vi "Version_2.0_Single_Column_Code.vi"() -> ()   [LabVIEW 2020] (continued)
                                n6258 = local read "Pause Elution"() -> (w6664:bool)
                                n6259 = case shown="True" w6664 {
                                tunnel: w6663 -> [w6675 _]
                                tunnel: w6671 -> [w6674 w6717]
                                tunnel: w6670 -> [w6673 _]
                                tunnel: w6669 -> [w6672 _]
                                frame False {
                                n6260 = stacked-sequence {
                                tunnel: w6675 -> [_ w6681]
                                tunnel: w6674 -> [_ w6680]
                                tunnel: w6673 -> [_ w6679]
                                tunnel: w6672 -> [_ w6678]
                                frame #0 {
                                n6261 = Wait (ms)(milliseconds to wait=u32 3000) -> ()  [unwired: 1 out]
                                n6262 = local write "Signal"(TRUE ("Signal")) -> ()
                                }
                                frame #1 {
                                n6263 = while {
                                tunnel: w6681 -> [w6693]
                                tunnel: w6680 -> [w6692]
                                tunnel: w6679 -> [w6691]
                                tunnel: w6678 -> [w6690]
                                stop <- w6685 stop-if-true
                                n6264 = stacked-sequence {
                                tunnel: w6693 -> [_ w6700]
                                tunnel: w6692 -> [_ w6699]
                                tunnel: w6691 -> [_ w6698]
                                tunnel: w6690 -> [_ w6697]
                                frame #0 {
                                n6265 = Wait (ms)(milliseconds to wait=u32 500) -> ()  [unwired: 1 out]
                                }
                                frame #1 {
                                n6266 = call "AbsolutePlungerPosition (SubVI).vi"("VISA Refnum in"=w6699) -> ("Plunger Position"=w6696:i32)  [unwired: 10 in]
                                n6267 = case shown="\"High Resolution Pumping\"" w6698 {
                                tunnel: w6700 -> [w6705 w6714]
                                tunnel: w6696 -> [w6706 w6713]
                                tunnel: [w6704 w6711] -> w6695
                                tunnel: w6697 -> [w6703 w6712]
                                frame "Standard Pumping", Default {
                                n6268 = Subtract(x=w6705, y=w6706) -> (x-y=w6702:dbl)
                                n6269 = Absolute Value(x=w6702) -> (abs(x)=w6701:dbl)
                                n6270 = Multiply(x=w6701, y=w6703) -> (x*y=w6708:dbl)
                                n6271 = Divide(x=w6708, y=3000.0) -> (x/y=w6704:dbl)
                                }
                                frame "High Resolution Pumping" {
                                n6272 = Subtract(x=w6714, y=w6713) -> (x-y=w6710:dbl)
                                n6273 = Absolute Value(x=w6710) -> (abs(x)=w6709:dbl)
                                n6274 = Multiply(x=w6709, y=w6712) -> (x*y=w6716:dbl)
                                n6275 = Divide(x=w6716, y=24000.0) -> (x/y=w6711:dbl)
                                }
                                }
                                n6276 = local write "Volume being Injected \nin this process"(w6695) -> ()
                                }
                                }
                                n6277 = local read "Volume being Injected \nin this process"() -> (w6683:dbl)
                                n6278 = local read "Affinity Elution \nGraph Min CutOff"() -> (w6682:dbl)
                                n6279 = local read "Stopper that ends \nthe main loops"() -> (w6688:bool)
                                n6280 = local read "Divert Sample \ninto Column-2"() -> (w6689:bool)
                                n6281 = Greater Or Equal?(x=w6683, y=w6682) -> (x >= y?=w6684:bool)
                                n6282 = Or(x=w6689, y=w6688) -> (x .or. y?=w6686:bool)
                                n6283 = local read "Pause Elution"() -> (w6687:bool)
                                n6284 = local write "Affinity Elution \nis Approaching"(w6684) -> ()
                                n6285 = Or(x=w6687, y=w6686) -> (x .or. y?=w6685:bool)
                                }
                                }
                                }
                                }
                                frame True {
                                n6286 = stacked-sequence {
                                tunnel: w6717 -> [_ w6720 _]
                                frame #0 {
                                n6287 = Wait (ms)(milliseconds to wait=u32 2000) -> ()  [unwired: 1 out]
                                }
                                frame #1 {
                                n6288 = local read "Signal"() -> (w6719:bool)
                                n6289 = case shown="True" w6719 {
                                tunnel: w6720 -> [_ w6726]
                                frame False {
                                }
                                frame True {
                                n6290 = local read "Volume being Injected \nin this process"() -> (w6724:dbl)
                                n6291 = local read "Net Elution \nVolume"() -> (w6723:dbl)
                                n6292 = local write "Signal"(FALSE ("Signal")) -> ()
                                n6293 = Add(x=w6724, y=w6723) -> (x+y=w6722:dbl)
                                n6294 = call "AbsolutePlungerPosition (SubVI).vi"("VISA Refnum in"=w6726) -> ("Plunger Position"=w6725:i32)  [unwired: 10 in]
                                n6295 = local write "Net Elution \nVolume"(w6722) -> ()
                                n6296 = local write "Position\nNow"(w6725) -> ()
                                }
                                }
                                }
                                frame #2 {
                                n6297 = local write "Volume being Injected \nin this process"(0.0 ("Volume being Injected \nin this process")) -> ()
                                }
                                }
                                }
                                }
                                n6298 = local read "Stopper that ends \nthe main loops"() -> (w6667:bool)
                                n6299 = local read "Divert Sample \ninto Column-2"() -> (w6666:bool)
                                n6300 = Or(x=w6666, y=w6667) -> (x .or. y?=w6665:bool)
                                n6301 = Wait (ms)(milliseconds to wait=u32 300) -> ()  [unwired: 1 out]
                                }
                                n6302 = local read "Stopper that ends \nthe main loops"() -> (w6643:bool)
                                n6303 = case shown="True" w6643 {
                                frame False {
                                }
                                frame True {
                                n6304 = local read "VISA Refnum in\nfor Pump"() -> (w6728:refnum<visa-resource-name>)
                                n6305 = call "HardStopCurrentProcess (SubVI).vi"("VISA Refnum in"=w6728) -> ()  [unwired: 11 in]
                                }
                                }
                                }
                                frame #15 {
                                # "valve after column-1 is closed"
                                # "Keeps the on-chip Valve V1 and V3 after column-2 open"
                                # "Keeps the AMF valve after column-1 closed and valve after column-2 open"
                                n6306 = local read "VISA Refnum in\nfor Pump"() -> (w6741:refnum<visa-resource-name>)
                                n6307 = local read "Volume being Injected \nin this process"() -> (w6738:dbl)
                                n6308 = local write "Sample Volume Diverted\ninto Column-2"(0.0 ("Sample Volume Diverted\ninto Column-2")) -> ()
                                n6309 = call "AbsolutePlungerPosition (SubVI).vi"("VISA Refnum in"=w6741) -> ("Plunger Position"=w6740:i32)  [unwired: 10 in]
                                n6310 = local write "Position\nNow"(w6740) -> ()
                                n6311 = local write "Vol_previous"(0.0 ("Vol_diff")) -> ()
                                n6312 = local write "Vol_now"(w6738) -> ()
                                n6313 = local read "VISA Refnum in\nfor Valve"() -> (w6733:refnum<visa-resource-name>)
                                n6314 = local read "External Valve \nCLOSED"() -> (w6732:string)
                                n6315 = local write "Valve V1 Open"(TRUE ("Valve V1 Open")) -> ()
                                n6316 = local write "Valve V3 Open"(TRUE ("Valve V3 Open")) -> ()
                                n6317 = local write "Valve V2 Open"(FALSE ("Valve V2 Open")) -> ()
                                n6318 = local write "Valve V4 Open"(TRUE ("Valve V4 Open")) -> ()
                                n6319 = call "PortChanger_Valve (SubVI).vi"("Port Number"=w6732, "VISA Refnum in"=w6733) -> ()  [unwired: 10 in]
                                n6320 = local write "Valve V5 Open"(TRUE ("Valve V5 Open")) -> ()
                                n6321 = local write "Valve V6 Open"(FALSE ("Valve V6 Open")) -> ()
                                n6322 = local write "Valve V7 Open"(TRUE ("Valve V7 Open")) -> ()
                                }
                                frame #16 {
                                n6323 = local read "Divert Sample \ninto Column-2"() -> (w6743:bool)
                                n6324 = case shown="True" w6743 {
                                frame False {
                                n6325 = stacked-sequence {
                                frame #0 {
                                n6326 = local read "Buffer-B Pumping\nResolution"() -> (w6746:T2)
                                n6327 = local read "VISA Refnum in\nfor Pump"() -> (w6748:refnum<visa-resource-name>)
                                n6328 = local read "Initial Plunger Position"() -> (w6747:dbl)
                                n6329 = local read "Volume of Syringe"() -> (w6745:dbl)
                                n6330 = while {
                                tunnel: w6747 -> [w6754]
                                tunnel: w6748 -> [w6753]
                                tunnel: w6746 -> [w6752]
                                tunnel: w6745 -> [w6751]
                                stop <- w6749 stop-if-true
                                n6331 = Wait (ms)(milliseconds to wait=u32 100) -> ()  [unwired: 1 out]
                                n6332 = stacked-sequence {
                                tunnel: w6754 -> [w6760 _]
                                tunnel: w6753 -> [w6759 w6780]
                                tunnel: w6752 -> [w6758 _]
                                tunnel: w6751 -> [w6757 _]
                                tunnel: [_ w6778] -> w6749
                                frame #0 {
                                n6333 = call "AbsolutePlungerPosition (SubVI).vi"("VISA Refnum in"=w6759) -> ("Plunger Position"=w6756:i32)  [unwired: 10 in]
                                n6334 = case shown="\"Standard Pumping\", Default" w6758 {
                                tunnel: w6760 -> [w6765 w6774]
                                tunnel: w6756 -> [w6766 w6773]
                                tunnel: [w6764 w6771] -> w6755
                                tunnel: w6757 -> [w6763 w6772]
                                frame "Standard Pumping", Default {
                                n6335 = Subtract(x=w6765, y=w6766) -> (x-y=w6762:dbl)
                                n6336 = Absolute Value(x=w6762) -> (abs(x)=w6761:dbl)
                                n6337 = Multiply(x=w6761, y=w6763) -> (x*y=w6768:dbl)
                                n6338 = Divide(x=w6768, y=3000.0) -> (x/y=w6764:dbl)
                                }
                                frame "High Resolution Pumping" {
                                n6339 = Subtract(x=w6774, y=w6773) -> (x-y=w6770:dbl)
                                n6340 = Absolute Value(x=w6770) -> (abs(x)=w6769:dbl)
                                n6341 = Multiply(x=w6769, y=w6772) -> (x*y=w6776:dbl)
                                n6342 = Divide(x=w6776, y=24000.0) -> (x/y=w6771:dbl)
                                }
                                }
                                n6343 = local write "Volume being Injected \nin this process"(w6755) -> ()
                                }
                                frame #1 {
                                n6344 = local read "Stopper that ends \nthe main loops"() -> (w6777:bool)
                                n6345 = call "LSPOneStatus (SubVI).vi"("VISA Refnum in"=w6780) -> ("read buffer"=w6782:string)  [unwired: 10 in]
                                n6346 = call <vilib>:"Trim Whitespace.vi"("string"=w6782) -> ("trimmed string"=w6781:string)  [unwired: 1 in]
                                n6347 = Equal?(x=w6781, y="/0`\u0003") -> (x = y?=w6779:bool)
                                n6348 = Or(x=w6779, y=w6777) -> (x .or. y?=w6778:bool)
                                }
                                }
                                }
                                n6349 = local read "Stopper that ends \nthe main loops"() -> (w6744:bool)
                                n6350 = case shown="True" w6744 {
                                frame False {
                                }
                                frame True {
                                n6351 = local read "VISA Refnum in\nfor Pump"() -> (w6784:refnum<visa-resource-name>)
                                n6352 = call "HardStopCurrentProcess (SubVI).vi"("VISA Refnum in"=w6784) -> ()  [unwired: 11 in]
                                }
                                }
                                }
                                }
                                }
                                frame True {
                                n6353 = stacked-sequence {
                                frame #0 {
                                n6354 = local read "Buffer-B Pumping\nResolution"() -> (w6787:T2)
                                n6355 = local read "VISA Refnum in\nfor Pump"() -> (w6789:refnum<visa-resource-name>)
                                n6356 = local read "Volume of Syringe"() -> (w6786:dbl)
                                n6357 = local read "Position\nNow"() -> (w6788:dbl)
                                n6358 = while {
                                tunnel: w6788 -> [w6795]
                                tunnel: w6789 -> [w6794]
                                tunnel: w6787 -> [w6793]
                                tunnel: w6786 -> [w6792]
                                stop <- w6790 stop-if-true
                                n6359 = Wait (ms)(milliseconds to wait=u32 100) -> ()  [unwired: 1 out]
                                n6360 = stacked-sequence {
                                tunnel: w6795 -> [w6805 _ _]
                                tunnel: w6794 -> [w6804 _ w6831]
                                tunnel: w6793 -> [w6803 _ _]
                                tunnel: w6792 -> [w6802 _ _]
                                tunnel: [_ _ w6829] -> w6790
                                frame #0 {
                                n6361 = local read "Vol_previous"() -> (w6799:dbl)
                                n6362 = call "AbsolutePlungerPosition (SubVI).vi"("VISA Refnum in"=w6804) -> ("Plunger Position"=w6801:i32)  [unwired: 10 in]
                                n6363 = case shown="\"Standard Pumping\", Default" w6803 {
                                tunnel: w6805 -> [w6810 w6819]
                                tunnel: w6801 -> [w6811 w6818]
                                tunnel: [w6809 w6816] -> w6800
                                tunnel: w6802 -> [w6808 w6817]
                                frame "Standard Pumping", Default {
                                n6364 = Subtract(x=w6810, y=w6811) -> (x-y=w6807:dbl)
                                n6365 = Absolute Value(x=w6807) -> (abs(x)=w6806:dbl)
                                n6366 = Multiply(x=w6806, y=w6808) -> (x*y=w6813:dbl)
                                n6367 = Divide(x=w6813, y=3000.0) -> (x/y=w6809:dbl)
                                }
                                frame "High Resolution Pumping" {
                                n6368 = Subtract(x=w6819, y=w6818) -> (x-y=w6815:dbl)
                                n6369 = Absolute Value(x=w6815) -> (abs(x)=w6814:dbl)
                                n6370 = Multiply(x=w6814, y=w6817) -> (x*y=w6821:dbl)
                                n6371 = Divide(x=w6821, y=24000.0) -> (x/y=w6816:dbl)
                                }
                                }
                                n6372 = Subtract(x=w6800, y=w6799) -> (x-y=w6798:dbl)
                                n6373 = local read "Vol_now"() -> (w6796:dbl)
                                n6374 = local write "Sample Volume Diverted\ninto Column-2"(w6800) -> ()
                                n6375 = Add(x=w6798, y=w6796) -> (x+y=w6797:dbl)
                                n6376 = local write "Volume being Injected \nin this process"(w6797) -> ()
                                }
                                frame #1 {
                                n6377 = local read "Volume being Injected \nin this process"() -> (w6822:dbl)
                                n6378 = local read "Sample Volume Diverted\ninto Column-2"() -> (w6823:dbl)
                                n6379 = local write "Vol_now"(w6822) -> ()
                                n6380 = local write "Vol_previous"(w6823) -> ()
                                }
                                frame #2 {
                                n6381 = local read "Buffer-B Volume \nto be Pumped for\nSample Diversion\nto Column-2"() -> (w6825:dbl)
                                n6382 = local read "Sample Volume Diverted\ninto Column-2"() -> (w6824:dbl)
                                n6383 = local read "Stopper that ends \nthe main loops"() -> (w6826:bool)
                                n6384 = call "LSPOneStatus (SubVI).vi"("VISA Refnum in"=w6831) -> ("read buffer"=w6833:string)  [unwired: 10 in]
                                n6385 = call <vilib>:"Trim Whitespace.vi"("string"=w6833) -> ("trimmed string"=w6832:string)  [unwired: 1 in]
                                n6386 = Equal?(x=w6832, y="/0`\u0003") -> (x = y?=w6830:bool)
                                n6387 = Greater Or Equal?(x=w6824, y=w6825) -> (x >= y?=w6828:bool)
                                n6388 = Or(x=w6826, y=w6828) -> (x .or. y?=w6827:bool)
                                n6389 = Or(x=w6830, y=w6827) -> (x .or. y?=w6829:bool)
                                }
                                }
                                }
                                n6390 = local read "Stopper that ends \nthe main loops"() -> (w6785:bool)
                                n6391 = case shown="True" w6785 {
                                frame False {
                                }
                                frame True {
                                n6392 = local read "VISA Refnum in\nfor Pump"() -> (w6835:refnum<visa-resource-name>)
                                n6393 = call "HardStopCurrentProcess (SubVI).vi"("VISA Refnum in"=w6835) -> ()  [unwired: 11 in]
                                }
                                }
                                }
                                frame #1 {
                                n6394 = local read "VISA Refnum in\nfor Pump"() -> (w6837:refnum<visa-resource-name>)
                                n6395 = local write "Pause Data Collection"(TRUE ("Pause Data Collection")) -> ()
                                n6396 = call "HardStopCurrentProcess (SubVI).vi"("VISA Refnum in"=w6837) -> ()  [unwired: 11 in]
                                }
                                frame #2 {
                                n6397 = local read "VISA Refnum in\nfor Pump"() -> (w6838:refnum<visa-resource-name>)
                                n6398 = call "PortChanger (SubVI).vi"("Port Number"="1", "VISA Refnum in"=w6838) -> ()  [unwired: 10 in]
                                }
                                frame #3 {
                                n6399 = local read "VISA Refnum in\nfor Pump"() -> (w6844:refnum<visa-resource-name>)
                                n6400 = local read "Volume of Syringe"() -> (w6840:dbl)
                                n6401 = call "GoToAbsolutePosition(SubVI).vi"("Absolute Volume Position in Syringe (in ul)"=0.0, "Volume of Syringe"=w6840, "Resolution of Pumping"=T2."Standard Pumping", "Flow Rate (ul/min)"=150.0, "VISA Refnum in"=w6844) -> ()  [unwired: 6 in, 1 out]
                                }
                                frame #4 {
                                n6402 = local read "VISA Refnum in\nfor Pump"() -> (w6846:refnum<visa-resource-name>)
                                n6403 = local write "Divert Sample \ninto Column-2"(FALSE ("Divert Sample \ninto Column-2")) -> ()
                                n6404 = call "ProcessCompletionWaiter (SubVI).vi"("VISA Refnum in"=w6846) -> ()  [unwired: 11 in]
                                }
                                }
                                }
                                }
                                }
                                frame #17 {
                                # "Keeps the On-Chip Valves V1 and V3 closed"
                                # "Switch to Port-5/8"
                                # "Port-5/8 of pump is connected to Buffer-C1/C2"
                                # "Keeps the AMF valve after column-1 open and valve after column-2 closed"
                                n6405 = local read "VISA Refnum in\nfor Pump"() -> (w6859:refnum<visa-resource-name>)
                                n6406 = local write "Pause Data Collection"(TRUE ("Pause Data Collection")) -> ()
                                n6407 = Wait (ms)(milliseconds to wait=u32 500) -> ()  [unwired: 1 out]
                                n6408 = local write "Affinity On"(FALSE ("Affinity On")) -> ()
                                n6409 = local read "Port for \nC2-Elution"() -> (w6850:string)
                                n6410 = local write "Affinity Elution On"(FALSE ("Affinity Elution On")) -> ()
                                n6411 = call "PortChanger (SubVI).vi"("Port Number"=w6850, "VISA Refnum in"=w6859) -> ()  [unwired: 10 in]
                                n6412 = local read "VISA Refnum in\nfor Valve"() -> (w6853:refnum<visa-resource-name>)
                                n6413 = local read "External Valve \nCLOSED"() -> (w6852:string)
                                n6414 = local write "Valve V1 Open"(FALSE ("Valve V1 Open")) -> ()
                                n6415 = local write "Valve V2 Open"(FALSE ("Valve V2 Open")) -> ()
                                n6416 = local write "Valve V3 Open"(FALSE ("Valve V3 Open")) -> ()
                                n6417 = local write "Valve V4 Open"(FALSE ("Valve V4 Open")) -> ()
                                n6418 = call "PortChanger_Valve (SubVI).vi"("Port Number"=w6852, "VISA Refnum in"=w6853) -> ()  [unwired: 10 in]
                                n6419 = local write "Valve V5 Open"(FALSE ("Valve V5 Open")) -> ()
                                n6420 = local write "Valve V6 Open"(FALSE ("Valve V6 Open")) -> ()
                                n6421 = local write "Valve V7 Open"(FALSE ("Valve V7 Open")) -> ()
                                }
                                frame #18 {
                                n6422 = local read "VISA Refnum in\nfor Pump"() -> (w6863:refnum<visa-resource-name>)
                                n6423 = call "ProcessCompletionWaiter (SubVI).vi"("VISA Refnum in"=w6863) -> ()  [unwired: 11 in]
                                n6424 = local write "Start the Process"(FALSE ("Start the Process")) -> ()
                                }
                                frame #19 {
                                n6425 = local read "Stopper that ends \nthe main loops"() -> (w6867:bool)
                                n6426 = local read "Start the Process"() -> (w6868:bool)
                                n6427 = Or(x=w6868, y=w6867) -> (x .or. y?=w6866:bool)
                                n6428 = local write "Elution of Column-1"(FALSE ("Elution of Column-1")) -> ()
                                n6429 = case shown="False" w6866 {
                                frame False {
                                n6430 = while {
                                stop <- w6872 stop-if-true
                                n6431 = local read "Stopper that ends \nthe main loops"() -> (w6873:bool)
                                n6432 = local read "Start the Process"() -> (w6874:bool)
                                n6433 = Or(x=w6874, y=w6873) -> (x .or. y?=w6872:bool)
                                n6434 = Wait (ms)(milliseconds to wait=u32 10) -> ()  [unwired: 1 out]
                                }
                                n6435 = One Button Dialog(message="Move to Column-2 detection zone and Press 'Start the Process' Button.") -> ()  [unwired: 1 in, 1 out]
                                }
                                frame True {
                                }
                                }
                                n6436 = local write "Volume being Injected \nin this process"(0.0 ("Volume being Injected \nin this process")) -> ()
                                n6437 = local write "Elution of Column-2"(TRUE ("Elution of Column-2")) -> ()
                                }
                                frame #20 {
                                # "If Yes, it will clean the SEC buffer from port-8 tubing else it will clean the pump valve a bit"
                                n6438 = local read "Clean the \nBuffer-C2 tubing"() -> (w6875:bool)
                                n6439 = case shown="False" w6875 {
                                frame False {
                                n6440 = stacked-sequence {
                                frame #0 {
                                n6441 = local read "VISA Refnum in\nfor Pump"() -> (w6877:refnum<visa-resource-name>)
                                n6442 = local read "Port for \nC2-Elution"() -> (w6876:string)
                                n6443 = call "PortChanger (SubVI).vi"("Port Number"=w6876, "VISA Refnum in"=w6877) -> ()  [unwired: 10 in]
                                }
                                frame #1 {
                                n6444 = local read "VISA Refnum in\nfor Pump"() -> (w6878:refnum<visa-resource-name>)
                                n6445 = call "ProcessCompletionWaiter (SubVI).vi"("VISA Refnum in"=w6878) -> ()  [unwired: 11 in]
                                }
                                frame #2 {
                                n6446 = local read "Buffer-C2 Pumping\nResolution"() -> (w6881:T2)
                                n6447 = local read "VISA Refnum in\nfor Pump"() -> (w6883:refnum<visa-resource-name>)
                                n6448 = local read "V-S"() -> (w6879:dbl)
                                n6449 = local read "Volume of Syringe"() -> (w6882:dbl)
                                n6450 = call "RPickUp(SubVI).vi"("Volume to be picked up"=w6879, "Volume of Syringe"=w6882, "Resolution of PickUP"=w6881, "PickUp Flow Rate (ul/min)"=150.0, "VISA Refnum in"=w6883) -> ()  [unwired: 6 in, 1 out]
                                }
                                frame #3 {
                                n6451 = local read "Stopper that ends \nthe main loops"() -> (w6884:bool)
                                n6452 = local read "VISA Refnum in\nfor Pump"() -> (w6885:refnum<visa-resource-name>)
                                n6453 = case shown="True" w6884 {
                                frame False {
                                }
                                frame True {
                                n6454 = local read "VISA Refnum in\nfor Pump"() -> (w6886:refnum<visa-resource-name>)
                                n6455 = call "HardStopCurrentProcess (SubVI).vi"("VISA Refnum in"=w6886) -> ()  [unwired: 11 in]
                                }
                                }
                                n6456 = call "ProcessCompletionWaiter (SubVI).vi"("VISA Refnum in"=w6885) -> ()  [unwired: 11 in]
                                }
                                frame #4 {
                                n6457 = local read "VISA Refnum in\nfor Pump"() -> (w6888:refnum<visa-resource-name>)
                                n6458 = call "PortChanger (SubVI).vi"("Port Number"="1", "VISA Refnum in"=w6888) -> ()  [unwired: 10 in]
                                }
                                frame #5 {
                                n6459 = local read "Stopper that ends \nthe main loops"() -> (w6889:bool)
                                n6460 = local read "VISA Refnum in\nfor Pump"() -> (w6890:refnum<visa-resource-name>)
                                n6461 = case shown="True" w6889 {
                                frame False {
                                }
                                frame True {
                                n6462 = local read "VISA Refnum in\nfor Pump"() -> (w6891:refnum<visa-resource-name>)
                                n6463 = call "HardStopCurrentProcess (SubVI).vi"("VISA Refnum in"=w6891) -> ()  [unwired: 11 in]
                                }
                                }
                                n6464 = call "ProcessCompletionWaiter (SubVI).vi"("VISA Refnum in"=w6890) -> ()  [unwired: 11 in]
                                }
                                frame #6 {
                                n6465 = local read "VISA Refnum in\nfor Pump"() -> (w6896:refnum<visa-resource-name>)
                                n6466 = local read "Volume of Syringe"() -> (w6893:dbl)
                                n6467 = call "GoToAbsolutePosition(SubVI).vi"("Absolute Volume Position in Syringe (in ul)"=0.0, "Volume of Syringe"=w6893, "Resolution of Pumping"=T2."Standard Pumping", "Flow Rate (ul/min)"=150.0, "VISA Refnum in"=w6896) -> ()  [unwired: 6 in, 1 out]
                                }
                                frame #7 {
                                n6468 = local read "Stopper that ends \nthe main loops"() -> (w6897:bool)
                                n6469 = local read "VISA Refnum in\nfor Pump"() -> (w6898:refnum<visa-resource-name>)
                                n6470 = case shown="True" w6897 {
                                frame False {
                                }
                                frame True {
                                n6471 = local read "VISA Refnum in\nfor Pump"() -> (w6899:refnum<visa-resource-name>)
                                n6472 = call "HardStopCurrentProcess (SubVI).vi"("VISA Refnum in"=w6899) -> ()  [unwired: 11 in]
                                }
                                }
                                n6473 = call "ProcessCompletionWaiter (SubVI).vi"("VISA Refnum in"=w6898) -> ()  [unwired: 11 in]
                                }
                                }
                                }
                                frame True {
                                n6474 = for {
                                N: 2 -> [_]
                                n6475 = stacked-sequence {
                                frame #0 {
                                n6476 = local read "VISA Refnum in\nfor Pump"() -> (w6902:refnum<visa-resource-name>)
                                n6477 = local read "Port for \nC2-Elution"() -> (w6901:string)
                                n6478 = call "PortChanger (SubVI).vi"("Port Number"=w6901, "VISA Refnum in"=w6902) -> ()  [unwired: 10 in]
                                }
                                frame #1 {
                                n6479 = local read "VISA Refnum in\nfor Pump"() -> (w6903:refnum<visa-resource-name>)
                                n6480 = call "ProcessCompletionWaiter (SubVI).vi"("VISA Refnum in"=w6903) -> ()  [unwired: 11 in]
                                }
                                frame #2 {
                                n6481 = local read "Buffer-C2 Pumping\nResolution"() -> (w6906:T2)
                                n6482 = local read "VISA Refnum in\nfor Pump"() -> (w6908:refnum<visa-resource-name>)
                                n6483 = local read "Apparent Volume\nof Syringe"() -> (w6904:dbl)
                                n6484 = local read "Volume of Syringe"() -> (w6907:dbl)
                                n6485 = call "RPickUp(SubVI).vi"("Volume to be picked up"=w6904, "Volume of Syringe"=w6907, "Resolution of PickUP"=w6906, "PickUp Flow Rate (ul/min)"=150.0, "VISA Refnum in"=w6908) -> ()  [unwired: 6 in, 1 out]
                                }
                                frame #3 {
                                n6486 = local read "Stopper that ends \nthe main loops"() -> (w6909:bool)
                                n6487 = local read "VISA Refnum in\nfor Pump"() -> (w6910:refnum<visa-resource-name>)
                                n6488 = case shown="True" w6909 {
                                frame False {
                                }
                                frame True {
                                n6489 = local read "VISA Refnum in\nfor Pump"() -> (w6911:refnum<visa-resource-name>)
                                n6490 = call "HardStopCurrentProcess (SubVI).vi"("VISA Refnum in"=w6911) -> ()  [unwired: 11 in]
                                }
                                }
                                n6491 = call "ProcessCompletionWaiter (SubVI).vi"("VISA Refnum in"=w6910) -> ()  [unwired: 11 in]
                                }
                                frame #4 {
                                n6492 = local read "VISA Refnum in\nfor Pump"() -> (w6913:refnum<visa-resource-name>)
                                n6493 = call "PortChanger (SubVI).vi"("Port Number"="1", "VISA Refnum in"=w6913) -> ()  [unwired: 10 in]
                                }
                                frame #5 {
                                n6494 = local read "Stopper that ends \nthe main loops"() -> (w6914:bool)
                                n6495 = local read "VISA Refnum in\nfor Pump"() -> (w6915:refnum<visa-resource-name>)
                                n6496 = case shown="True" w6914 {
                                frame False {
                                }
                                frame True {
                                n6497 = local read "VISA Refnum in\nfor Pump"() -> (w6916:refnum<visa-resource-name>)
                                n6498 = call "HardStopCurrentProcess (SubVI).vi"("VISA Refnum in"=w6916) -> ()  [unwired: 11 in]
                                }
                                }
                                n6499 = call "ProcessCompletionWaiter (SubVI).vi"("VISA Refnum in"=w6915) -> ()  [unwired: 11 in]
                                }
                                frame #6 {
                                n6500 = local read "VISA Refnum in\nfor Pump"() -> (w6921:refnum<visa-resource-name>)
                                n6501 = local read "Volume of Syringe"() -> (w6918:dbl)
                                n6502 = call "GoToAbsolutePosition(SubVI).vi"("Absolute Volume Position in Syringe (in ul)"=0.0, "Volume of Syringe"=w6918, "Resolution of Pumping"=T2."Standard Pumping", "Flow Rate (ul/min)"=150.0, "VISA Refnum in"=w6921) -> ()  [unwired: 6 in, 1 out]
                                }
                                frame #7 {
                                n6503 = local read "Stopper that ends \nthe main loops"() -> (w6922:bool)
                                n6504 = local read "VISA Refnum in\nfor Pump"() -> (w6923:refnum<visa-resource-name>)
                                n6505 = case shown="True" w6922 {
                                frame False {
                                }
                                frame True {
                                n6506 = local read "VISA Refnum in\nfor Pump"() -> (w6924:refnum<visa-resource-name>)
                                n6507 = call "HardStopCurrentProcess (SubVI).vi"("VISA Refnum in"=w6924) -> ()  [unwired: 11 in]
                                }
                                }
                                n6508 = call "ProcessCompletionWaiter (SubVI).vi"("VISA Refnum in"=w6923) -> ()  [unwired: 11 in]
                                }
                                }
                                }
                                }
                                }
                                }
                                frame #21 {
                                n6509 = local read "VISA Refnum in\nfor Pump"() -> (w6926:refnum<visa-resource-name>)
                                n6510 = local read "Port for \nC2-Elution"() -> (w6925:string)
                                n6511 = call "PortChanger (SubVI).vi"("Port Number"=w6925, "VISA Refnum in"=w6926) -> ()  [unwired: 10 in]
                                }
                                frame #22 {
                                n6512 = local read "VISA Refnum in\nfor Pump"() -> (w6927:refnum<visa-resource-name>)
                                n6513 = call "ProcessCompletionWaiter (SubVI).vi"("VISA Refnum in"=w6927) -> ()  [unwired: 11 in]
                                }
                                frame #23 {
                                n6514 = local read "Buffer-C2 PickUp \nFlow Rate (ul/min)"() -> (w6931:dbl)
                                n6515 = local read "Buffer-C2 Pumping\nResolution"() -> (w6930:T2)
                                n6516 = local read "VISA Refnum in\nfor Pump"() -> (w6933:refnum<visa-resource-name>)
                                n6517 = local read "Buffer-C2 Volume \nto be Pumped"() -> (w6929:dbl)
                                n6518 = local read "Volume of Syringe"() -> (w6932:dbl)
                                n6519 = call "RPickUp(SubVI).vi"("Volume to be picked up"=w6929, "Volume of Syringe"=w6932, "Resolution of PickUP"=w6930, "PickUp Flow Rate (ul/min)"=w6931, "VISA Refnum in"=w6933) -> ()  [unwired: 6 in, 1 out]
                                n6520 = local write "SEC On"(TRUE ("SEC On")) -> ()
                                }
                                frame #24 {
                                n6521 = local read "Stopper that ends \nthe main loops"() -> (w6934:bool)
                                n6522 = local read "VISA Refnum in\nfor Pump"() -> (w6935:refnum<visa-resource-name>)
                                n6523 = case shown="True" w6934 {
                                frame False {
                                }
                                frame True {
                                n6524 = local read "VISA Refnum in\nfor Pump"() -> (w6936:refnum<visa-resource-name>)
                                n6525 = call "HardStopCurrentProcess (SubVI).vi"("VISA Refnum in"=w6936) -> ()  [unwired: 11 in]
                                }
                                }
                                n6526 = call "ProcessCompletionWaiter (SubVI).vi"("VISA Refnum in"=w6935) -> ()  [unwired: 11 in]
                                }
                                frame #25 {
                                # "Reads the initial Plunger Position for computing the volume dispensed"
                                n6527 = local read "VISA Refnum in\nfor Pump"() -> (w6938:refnum<visa-resource-name>)
                                n6528 = call "AbsolutePlungerPosition (SubVI).vi"("VISA Refnum in"=w6938) -> ("Plunger Position"=w6937:i32)  [unwired: 10 in]
                                n6529 = local write "Initial Plunger Position"(w6937) -> ()
                                }
                                frame #26 {
                                # "Switch to Port-10"
                                # "Port-10 of the pump is conncted to column-2 of chip"
                                n6530 = local read "VISA Refnum in\nfor Pump"() -> (w6940:refnum<visa-resource-name>)
                                n6531 = call "PortChanger (SubVI).vi"("Port Number"="10", "VISA Refnum in"=w6940) -> ()  [unwired: 10 in]
                                }
                                frame #27 {
                                n6532 = local read "Stopper that ends \nthe main loops"() -> (w6941:bool)
                                n6533 = local read "VISA Refnum in\nfor Pump"() -> (w6942:refnum<visa-resource-name>)
                                n6534 = call "ProcessCompletionWaiter (SubVI).vi"("VISA Refnum in"=w6942) -> ()  [unwired: 11 in]
                                n6535 = case shown="True" w6941 {
                                frame False {
                                }
                                frame True {
                                n6536 = local read "VISA Refnum in\nfor Pump"() -> (w6943:refnum<visa-resource-name>)
                                n6537 = call "HardStopCurrentProcess (SubVI).vi"("VISA Refnum in"=w6943) -> ()  [unwired: 11 in]
                                }
                                }
                                }
                                frame #28 {
                                # "Keeps the AMF valve after column-1 open and valve after column-2 closed"
                                n6538 = local read "Buffer-C2 Dispense\nFlow Rate (ul/min)"() -> (w6956:dbl)
                                n6539 = local read "Buffer-C2 Pumping\nResolution"() -> (w6955:T2)
                                n6540 = local read "VISA Refnum in\nfor Pump"() -> (w6958:refnum<visa-resource-name>)
                                n6541 = local write "Pause Data Collection"(FALSE ("Pause Data Collection")) -> ()
                                n6542 = local read "Volume of Syringe"() -> (w6957:dbl)
                                n6543 = call "GoToAbsolutePosition(SubVI).vi"("Absolute Volume Position in Syringe (in ul)"=0.0 ("Volume to be Dispensed"), "Volume of Syringe"=w6957, "Resolution of Pumping"=w6955, "Flow Rate (ul/min)"=w6956, "VISA Refnum in"=w6958) -> ()  [unwired: 6 in, 1 out]
                                n6544 = local read "VISA Refnum in\nfor Valve"() -> (w6952:refnum<visa-resource-name>)
                                n6545 = local read "External Valve \nOPEN"() -> (w6951:string)
                                n6546 = local write "Valve V1 Open"(FALSE ("Valve V1 Open")) -> ()
                                n6547 = local write "Valve V2 Open"(TRUE ("Valve V2 Open")) -> ()
                                n6548 = local write "Valve V3 Open"(TRUE ("Valve V3 Open")) -> ()
                                n6549 = local write "Valve V4 Open"(FALSE ("Valve V4 Open")) -> ()
                                n6550 = call "PortChanger_Valve (SubVI).vi"("Port Number"=w6951, "VISA Refnum in"=w6952) -> ()  [unwired: 10 in]
                                n6551 = local write "Valve V5 Open"(FALSE ("Valve V5 Open")) -> ()
                                n6552 = local write "Valve V6 Open"(FALSE ("Valve V6 Open")) -> ()
                                n6553 = local write "Valve V7 Open"(FALSE ("Valve V7 Open")) -> ()
                                }
                                frame #29 {
                                n6554 = local read "Initial Plunger Position"() -> (w6962:dbl)
                                n6555 = local read "Buffer-C2 Pumping\nResolution"() -> (w6961:T2)
                                n6556 = local read "VISA Refnum in\nfor Pump"() -> (w6963:refnum<visa-resource-name>)
                                n6557 = local read "Volume of Syringe"() -> (w6960:dbl)
                                n6558 = while {
                                tunnel: w6962 -> [w6969]
                                tunnel: w6963 -> [w6968]
                                tunnel: w6961 -> [w6967]
                                tunnel: w6960 -> [w6966]
                                stop <- w6964 stop-if-true
                                n6559 = Wait (ms)(milliseconds to wait=u32 100) -> ()  [unwired: 1 out]
                                n6560 = stacked-sequence {
                                tunnel: w6969 -> [w6975 _]
                                tunnel: w6968 -> [w6974 w7001]
                                tunnel: w6967 -> [w6973 _]
                                tunnel: w6966 -> [w6972 _]
                                tunnel: [_ w6997] -> w6964
                                frame #0 {
                                n6561 = call "AbsolutePlungerPosition (SubVI).vi"("VISA Refnum in"=w6974) -> ("Plunger Position"=w6971:i32)  [unwired: 10 in]
                                n6562 = case shown="\"Standard Pumping\", Default" w6973 {
                                tunnel: w6975 -> [w6980 w6989]
                                tunnel: w6971 -> [w6981 w6988]
                                tunnel: [w6979 w6986] -> w6970
                                tunnel: w6972 -> [w6978 w6987]
                                frame "Standard Pumping", Default {
                                n6563 = Subtract(x=w6980, y=w6981) -> (x-y=w6977:dbl)
                                n6564 = Absolute Value(x=w6977) -> (abs(x)=w6976:dbl)
                                n6565 = Multiply(x=w6976, y=w6978) -> (x*y=w6983:dbl)
                                n6566 = Divide(x=w6983, y=3000.0) -> (x/y=w6979:dbl)
                                }
                                frame "High Resolution Pumping" {
                                n6567 = Subtract(x=w6989, y=w6988) -> (x-y=w6985:dbl)
                                n6568 = Absolute Value(x=w6985) -> (abs(x)=w6984:dbl)
                                n6569 = Multiply(x=w6984, y=w6987) -> (x*y=w6991:dbl)
                                n6570 = Divide(x=w6991, y=24000.0) -> (x/y=w6986:dbl)
                                }
                                }
                                n6571 = local write "Volume being Injected \nin this process"(w6970) -> ()
                                }
                                frame #1 {
                                n6572 = local read "Stopper that ends \nthe main loops"() -> (w6998:bool)
                                n6573 = local read "Divert Buffer-C \ninto Column-2"() -> (w6999:bool)
                                n6574 = local read "Volume being Injected \nin this process"() -> (w6996:dbl)
                                n6575 = call "LSPOneStatus (SubVI).vi"("VISA Refnum in"=w7001) -> ("read buffer"=w7003:string)  [unwired: 10 in]
                                n6576 = call <vilib>:"Trim Whitespace.vi"("string"=w7003) -> ("trimmed string"=w7002:string)  [unwired: 1 in]
                                n6577 = Equal?(x=w7002, y="/0`\u0003") -> (x = y?=w7000:bool)
                                n6578 = Or(x=w6999, y=w6998) -> (x .or. y?=w6994:bool)
                                n6579 = Greater Or Equal?(x=w6996, y=2.0) -> (x >= y?=w6993:bool)
                                n6580 = Or(x=w6994, y=w6993) -> (x .or. y?=w6992:bool)
                                n6581 = Or(x=w7000, y=w6992) -> (x .or. y?=w6997:bool)
                                }
                                }
                                }
                                n6582 = local read "Stopper that ends \nthe main loops"() -> (w6959:bool)
                                n6583 = case shown="True" w6959 {
                                frame False {
                                }
                                frame True {
                                n6584 = local read "VISA Refnum in\nfor Pump"() -> (w7005:refnum<visa-resource-name>)
                                n6585 = call "HardStopCurrentProcess (SubVI).vi"("VISA Refnum in"=w7005) -> ()  [unwired: 11 in]
                                }
                                }
                                }
                                frame #30 {
                                # "Keeps the on-chip valves V4, V5 and V7 open"
                                # "Keeps the AMF valve after column-1 closed and valve after column-2 open"
                                n6586 = local write "Divert Buffer-C \ninto Column-2"(FALSE ("Divert Buffer-C \ninto Column-2")) -> ()
                                n6587 = local read "VISA Refnum in\nfor Pump"() -> (w7010:refnum<visa-resource-name>)
                                n6588 = local read "External Valve \nCLOSED"() -> (w7009:string)
                                n6589 = local write "Valve V3 Open"(FALSE ("Valve V3 Open")) -> ()
                                n6590 = local write "Valve V2 Open"(FALSE ("Valve V2 Open")) -> ()
                                n6591 = local write "Valve V1 Open"(FALSE ("Valve V1 Open")) -> ()
                                n6592 = local write "Valve V4 Open"(TRUE ("Valve V4 Open")) -> ()
                                n6593 = call "PortChanger_Valve (SubVI).vi"("Port Number"=w7009, "VISA Refnum in"=w7010) -> ()  [unwired: 10 in]
                                n6594 = local write "Valve V5 Open"(TRUE ("Valve V5 Open")) -> ()
                                n6595 = local write "Valve V6 Open"(FALSE ("Valve V6 Open")) -> ()
                                n6596 = local write "Valve V7 Open"(TRUE ("Valve V7 Open")) -> ()
                                }
                                frame #31 {
                                n6597 = local read "Initial Plunger Position"() -> (w7019:dbl)
                                n6598 = local read "Buffer-C2 Pumping\nResolution"() -> (w7018:T2)
                                n6599 = local read "VISA Refnum in\nfor Pump"() -> (w7020:refnum<visa-resource-name>)
                                n6600 = local read "Volume of Syringe"() -> (w7017:dbl)
                                n6601 = while {
                                tunnel: w7019 -> [w7026]
                                tunnel: w7020 -> [w7025]
                                tunnel: w7018 -> [w7024]
                                tunnel: w7017 -> [w7023]
                                stop <- w7021 stop-if-true
                                n6602 = Wait (ms)(milliseconds to wait=u32 100) -> ()  [unwired: 1 out]
                                n6603 = stacked-sequence {
                                tunnel: w7026 -> [w7032 _]
                                tunnel: w7025 -> [w7031 w7054]
                                tunnel: w7024 -> [w7030 _]
                                tunnel: w7023 -> [w7029 _]
                                tunnel: [_ w7052] -> w7021
                                frame #0 {
                                n6604 = call "AbsolutePlungerPosition (SubVI).vi"("VISA Refnum in"=w7031) -> ("Plunger Position"=w7028:i32)  [unwired: 10 in]
                                n6605 = case shown="\"Standard Pumping\", Default" w7030 {
                                tunnel: w7032 -> [w7037 w7046]
                                tunnel: w7028 -> [w7038 w7045]
                                tunnel: [w7036 w7043] -> w7027
                                tunnel: w7029 -> [w7035 w7044]
                                frame "Standard Pumping", Default {
                                n6606 = Subtract(x=w7037, y=w7038) -> (x-y=w7034:dbl)
                                n6607 = Absolute Value(x=w7034) -> (abs(x)=w7033:dbl)
                                n6608 = Multiply(x=w7033, y=w7035) -> (x*y=w7040:dbl)
                                n6609 = Divide(x=w7040, y=3000.0) -> (x/y=w7036:dbl)
                                }
                                frame "High Resolution Pumping" {
                                n6610 = Subtract(x=w7046, y=w7045) -> (x-y=w7042:dbl)
                                n6611 = Absolute Value(x=w7042) -> (abs(x)=w7041:dbl)
                                n6612 = Multiply(x=w7041, y=w7044) -> (x*y=w7048:dbl)
                                n6613 = Divide(x=w7048, y=24000.0) -> (x/y=w7043:dbl)
                                }
                                }
                                n6614 = local write "Volume being Injected \nin this process"(w7027) -> ()
                                }
                                frame #1 {
                                n6615 = call "LSPOneStatus (SubVI).vi"("VISA Refnum in"=w7054) -> ("read buffer"=w7056:string)  [unwired: 10 in]
                                n6616 = call <vilib>:"Trim Whitespace.vi"("string"=w7056) -> ("trimmed string"=w7055:string)  [unwired: 1 in]
                                n6617 = Equal?(x=w7055, y="/0`\u0003") -> (x = y?=w7053:bool)
                                n6618 = local read "Stopper that ends \nthe main loops"() -> (w7050:bool)
                                n6619 = local read "Divert Sample \nonto Grid"() -> (w7051:bool)
                                n6620 = Or(x=w7051, y=w7050) -> (x .or. y?=w7049:bool)
                                n6621 = Or(x=w7053, y=w7049) -> (x .or. y?=w7052:bool)
                                }
                                }
                                }
                                n6622 = local read "Stopper that ends \nthe main loops"() -> (w7016:bool)
                                n6623 = case shown="True" w7016 {
                                frame False {
                                }
                                frame True {
                                n6624 = local read "VISA Refnum in\nfor Pump"() -> (w7058:refnum<visa-resource-name>)
                                n6625 = call "HardStopCurrentProcess (SubVI).vi"("VISA Refnum in"=w7058) -> ()  [unwired: 11 in]
                                }
                                }
                                }
                                frame #32 {
                                n6626 = local read "Volume being Injected \nin this process"() -> (w7061:dbl)
                                n6627 = local read "VISA Refnum in\nfor Pump"() -> (w7063:refnum<visa-resource-name>)
                                n6628 = call "AbsolutePlungerPosition (SubVI).vi"("VISA Refnum in"=w7063) -> ("Plunger Position"=w7062:i32)  [unwired: 10 in]
                                n6629 = local write "Pause Data Collection"(TRUE) -> ()
                                n6630 = local write "True Volume being \ninjected in this\nprocess"(w7061) -> ()
                                n6631 = local write "Position\nNow"(w7062) -> ()
                                n6632 = Wait (ms)(milliseconds to wait=u32 500) -> ()  [unwired: 1 out]
                                }
                                frame #33 {
                                # "Sample Deposition onto EM-Grid"
                                n6633 = local read "Divert Sample \nonto Grid"() -> (w7064:bool)
                                n6634 = case shown="True" w7064 {
                                frame False {
                                }
                                frame True {
                                n6635 = stacked-sequence {
                                frame #0 {
                                # "Discard the initial volume of fluid that is present in the channel prior to detection"
                                n6636 = local read "Buffer-C2 Pumping\nResolution"() -> (w7075:T2)
                                n6637 = local read "Initial Plunger Position"() -> (w7074:dbl)
                                n6638 = local read "VISA Refnum in\nfor Pump"() -> (w7076:refnum<visa-resource-name>)
                                n6639 = local read "Position\nNow"() -> (w7072:dbl)
                                n6640 = local read "Volume of Syringe"() -> (w7073:dbl)
                                n6641 = local write "Pause Data Collection"(FALSE) -> ()
                                n6642 = while {
                                tunnel: w7076 -> [w7086]
                                tunnel: w7075 -> [w7085]
                                tunnel: w7074 -> [w7081]
                                tunnel: w7073 -> [w7084]
                                tunnel: w7072 -> [w7080]
                                stop <- w7082 stop-if-true
                                n6643 = stacked-sequence {
                                tunnel: w7086 -> [w7092 w7114 w7146]
                                tunnel: w7085 -> [w7091 w7113 _]
                                tunnel: w7081 -> [w7089 _ _]
                                tunnel: w7084 -> [w7088 w7111 _]
                                tunnel: [_ _ w7140] -> w7082
                                tunnel: w7080 -> [_ w7109 _]
                                frame #0 {
                                # "From here on 'True Volume being injected \nin this process' represents the true total \nvolume in this process"
                                n6644 = call "AbsolutePlungerPosition (SubVI).vi"("VISA Refnum in"=w7092) -> ("Plunger Position"=w7090:i32)  [unwired: 10 in]
                                n6645 = case shown="..\"Standard Pumping\"" w7091 {
                                tunnel: w7090 -> [w7100 w7108]
                                tunnel: w7089 -> [w7099 w7107]
                                tunnel: w7088 -> [w7096 w7104]
                                tunnel: [w7093 w7101] -> w7087
                                frame .."Standard Pumping" {
                                n6646 = Subtract(x=w7100, y=w7099) -> (x-y=w7098:dbl)
                                n6647 = Absolute Value(x=w7098) -> (abs(x)=w7097:dbl)
                                n6648 = Multiply(x=w7097, y=w7096) -> (x*y=w7095:dbl)
                                n6649 = Divide(x=w7095, y=3000.0) -> (x/y=w7093:dbl)
                                }
                                frame "High Resolution Pumping".. {
                                n6650 = Subtract(x=w7108, y=w7107) -> (x-y=w7106:dbl)
                                n6651 = Absolute Value(x=w7106) -> (abs(x)=w7105:dbl)
                                n6652 = Multiply(x=w7105, y=w7104) -> (x*y=w7103:dbl)
                                n6653 = Divide(x=w7103, y=24000.0) -> (x/y=w7101:dbl)
                                }
                                }
                                n6654 = local write "True Volume being \ninjected in this\nprocess"(w7087) -> ()
                                }
                                frame #1 {
                                # "From here on 'Volume being injected \nin this process' represents the volume \nin this sub process"
                                n6655 = call "AbsolutePlungerPosition (SubVI).vi"("VISA Refnum in"=w7114) -> ("Plunger Position"=w7112:i32)  [unwired: 10 in]
                                n6656 = case shown="..\"Standard Pumping\"" w7113 {
                                tunnel: w7112 -> [w7122 w7130]
                                tunnel: w7109 -> [w7121 w7129]
                                tunnel: w7111 -> [w7118 w7126]
                                tunnel: [w7115 w7123] -> w7110
                                frame .."Standard Pumping" {
                                n6657 = Subtract(x=w7122, y=w7121) -> (x-y=w7120:dbl)
                                n6658 = Absolute Value(x=w7120) -> (abs(x)=w7119:dbl)
                                n6659 = Multiply(x=w7119, y=w7118) -> (x*y=w7117:dbl)
                                n6660 = Divide(x=w7117, y=3000.0) -> (x/y=w7115:dbl)
                                }
                                frame "High Resolution Pumping".. {
                                n6661 = Subtract(x=w7130, y=w7129) -> (x-y=w7128:dbl)
                                n6662 = Absolute Value(x=w7128) -> (abs(x)=w7127:dbl)
                                n6663 = Multiply(x=w7127, y=w7126) -> (x*y=w7125:dbl)
                                n6664 = Divide(x=w7125, y=24000.0) -> (x/y=w7123:dbl)
                                }
                                }
                                n6665 = local write "Volume being Injected \nin this process"(w7110) -> ()
                                }
                                frame #2 {
                                n6666 = local read "Discard Volume"() -> (w7134:dbl)
                                n6667 = local read "Discard fluid \nprior to 1st \ndeposition"() -> (w7139:bool)
                                n6668 = local read "Volume being Injected \nin this process"() -> (w7138:dbl)
                                n6669 = Greater Or Equal?(x=w7138, y=w7134) -> (x >= y?=w7136:bool)
                                n6670 = call "AbsolutePlungerPositionStatus (SubVI).vi"("VISA Refnum in"=w7146) -> ("read buffer"=w7145:string)  [unwired: 10 in]
                                n6671 = local read "Stop for End of \nExperiment \nand Data Writing"() -> (w7132:bool)
                                n6672 = call <vilib>:"Trim Whitespace.vi"("string"=w7145) -> ("trimmed string"=w7144:string)  [unwired: 1 in]
                                n6673 = Not(x=w7139) -> (.not. x?=w7137:bool)
                                n6674 = Equal?(x=w7144, y="/0`\u0003") -> (x = y?=w7142:bool)
                                n6675 = Or(x=w7137, y=w7136) -> (x .or. y?=w7135:bool)
                                n6676 = local read "Re-SEC"() -> (w7133:bool)
                                n6677 = Or(x=w7132, y=w7133) -> (x .or. y?=w7131:bool)
                                n6678 = Or(x=w7135, y=w7131) -> (x .or. y?=w7141:bool)
                                n6679 = Or(x=w7142, y=w7141) -> (x .or. y?=w7140:bool)
                                }
                                }
                                n6680 = Wait (ms)(milliseconds to wait=u32 100) -> ()  [unwired: 1 out]
                                }
                                n6681 = local write "Valve V4 Open"(TRUE ("Valve V4 Open")) -> ()
                                n6682 = local write "Valve V3 Open"(FALSE ("Valve V3 Open")) -> ()
                                n6683 = local write "Valve V2 Open"(FALSE ("Valve V2 Open")) -> ()
                                n6684 = local write "Valve V1 Open"(FALSE ("Valve V1 Open")) -> ()
                                n6685 = local write "Valve V5 Open"(TRUE ("Valve V5 Open")) -> ()
                                n6686 = local write "Valve V6 Open"(TRUE ("Valve V6 Open")) -> ()
                                n6687 = local write "Valve V7 Open"(FALSE ("Valve V7 Open")) -> ()
                                n6688 = local write "Volume being Injected \nin this process"(0.0) -> ()
                                }
                                frame #1 {
                                # "Keeps the on-chip valve V1, V2 and V3 closed,\nHalts also deposition onto the grid\nand waits for the 1st redeposit command. Once the command is issued\nit starts pumpoing and moves onto the next frame"
                                n6689 = stacked-sequence {
                                frame #0 {
                                n6690 = local write "Valve V5 Open"(FALSE ("Valve V5 Open")) -> ()
                                n6691 = local write "Valve V1 Open"(FALSE ("Valve V1 Open")) -> ()
                                n6692 = local read "VISA Refnum in\nfor Pump"() -> (w7156:refnum<visa-resource-name>)
                                n6693 = local write "Valve V2 Open"(FALSE ("Valve V2 Open")) -> ()
                                n6694 = local write "Valve V6 Open"(FALSE ("Valve V6 Open")) -> ()
                                n6695 = local write "Re-deposit Sample\nonto Grid"(FALSE ("Redeposit Sample\nonto Grid")) -> ()
                                n6696 = local write "Pause Data Collection"(TRUE ("Pause Data Collection")) -> ()
                                n6697 = call "HardStopCurrentProcess (SubVI).vi"("VISA Refnum in"=w7156) -> ()  [unwired: 11 in]
                                n6698 = local write "Valve V7 Open"(FALSE ("Valve V7 Open")) -> ()
                                n6699 = local write "Valve V3 Open"(FALSE ("Valve V3 Open")) -> ()
                                n6700 = local write "Valve V4 Open"(FALSE ("Valve V4 Open")) -> ()
                                }
                                frame #1 {
                                n6701 = while {
                                stop <- w7162 stop-if-true
                                n6702 = local read "Stop for End of \nExperiment \nand Data Writing"() -> (w7160:bool)
                                n6703 = local read "Re-deposit Sample\nonto Grid"() -> (w7163:bool)
                                n6704 = local read "Re-SEC"() -> (w7161:bool)
                                n6705 = Or(x=w7160, y=w7161) -> (x .or. y?=w7159:bool)
                                n6706 = Or(x=w7163, y=w7159) -> (x .or. y?=w7162:bool)
                                }
                                n6707 = local write "Discard fluid \nprior to 1st \ndeposition"(FALSE ("Discard fluid \nprior to 1st \ndeposition")) -> ()
                                n6708 = One Button Dialog(message="Do you want to deposit sample on another grid? If yes, turn on 'Re-deposit Sample onto Grid'. Else turn on Re-SEC to do SEC again or STOP to end the experiment") -> ()  [unwired: 1 in, 1 out]
                                }
                                frame #2 {
                                n6709 = local write "Valve V6 Open"(TRUE ("Valve V3 Open")) -> ()
                                n6710 = local write "Valve V4 Open"(TRUE ("Valve V1 Open")) -> ()
                                n6711 = local write "Valve V5 Open"(TRUE ("Valve V2 Open")) -> ()
                                n6712 = local write "Valve V7 Open"(FALSE ("Valve V7 Open")) -> ()
                                }
                                frame #3 {
                                n6713 = local read "Re-deposit Sample\nonto Grid"() -> (w7168:bool)
                                n6714 = case shown="True" w7168 {
                                frame False {
                                n6715 = local write "Suction On/Off"(FALSE ("Suction On/Off")) -> ()
                                }
                                frame True {
                                n6716 = stacked-sequence {
                                frame #0 {
                                n6717 = local read "VISA Refnum in\nfor Pump"() -> (w7171:refnum<visa-resource-name>)
                                n6718 = call "AbsolutePlungerPosition (SubVI).vi"("VISA Refnum in"=w7171) -> ("Plunger Position"=w7170:i32)  [unwired: 10 in]
                                n6719 = local write "Position\nNow"(w7170) -> ()
                                }
                                frame #1 {
                                n6720 = local read "Buffer-C2 Pumping\nResolution"() -> (w7173:T2)
                                n6721 = case shown="\"Standard Pumping\", Default" w7173 {
                                tunnel: [w7174 w7185] -> w7172
                                frame "Standard Pumping", Default {
                                n6722 = local read "Buffer-C2 Volume \nto be Pumped"() -> (w7177:dbl)
                                n6723 = local read "Volume of Syringe"() -> (w7180:dbl)
                                n6724 = local read "Initial Plunger Position"() -> (w7184:dbl)
                                n6725 = local read "Position\nNow"() -> (w7183:dbl)
                                n6726 = Subtract(x=w7184, y=w7183) -> (x-y=w7182:dbl)
                                n6727 = Absolute Value(x=w7182) -> (abs(x)=w7181:dbl)
                                n6728 = Multiply(x=w7181, y=w7180) -> (x*y=w7179:dbl)
                                n6729 = Divide(x=w7179, y=3000.0) -> (x/y=w7176:dbl)
                                n6730 = Subtract(x=w7176, y=w7177) -> (x-y=w7175:dbl)
                                n6731 = Absolute Value(x=w7175) -> (abs(x)=w7174:dbl)
                                }
                                frame "High Resolution Pumping" {
                                n6732 = local read "Buffer-C2 Volume \nto be Pumped"() -> (w7188:dbl)
                                n6733 = local read "Volume of Syringe"() -> (w7191:dbl)
                                n6734 = local read "Initial Plunger Position"() -> (w7195:dbl)
                                n6735 = local read "Position\nNow"() -> (w7194:dbl)
                                n6736 = Subtract(x=w7195, y=w7194) -> (x-y=w7193:dbl)
                                n6737 = Absolute Value(x=w7193) -> (abs(x)=w7192:dbl)
                                n6738 = Multiply(x=w7192, y=w7191) -> (x*y=w7190:dbl)
                                n6739 = Divide(x=w7190, y=24000.0) -> (x/y=w7187:dbl)
                                n6740 = Subtract(x=w7187, y=w7188) -> (x-y=w7186:dbl)
                                n6741 = Absolute Value(x=w7186) -> (abs(x)=w7185:dbl)
                                }
                                }
                                n6742 = local write "Buffer-C Volume\nleft to be Pumped"(w7172) -> ()
                                }
                                frame #2 {
                                n6743 = local read "Buffer-C2 Dispense\nFlow Rate (ul/min)"() -> (w7199:dbl)
                                n6744 = local read "Buffer-C2 Pumping\nResolution"() -> (w7198:T2)
                                n6745 = local read "VISA Refnum in\nfor Pump"() -> (w7201:refnum<visa-resource-name>)
                                n6746 = local read "Volume of Syringe"() -> (w7200:dbl)
                                n6747 = call "GoToAbsolutePosition(SubVI).vi"("Absolute Volume Position in Syringe (in ul)"=0.0, "Volume of Syringe"=w7200, "Resolution of Pumping"=w7198, "Flow Rate (ul/min)"=w7199, "VISA Refnum in"=w7201) -> ()  [unwired: 6 in, 1 out]
                                n6748 = local write "Suction On/Off"(FALSE ("Suction On/Off")) -> ()
                                }
                                }
                                }
                                }
                                }
                                frame #4 {
                                n6749 = local read "Stop for End of \nExperiment \nand Data Writing"() -> (w7203:bool)
                                n6750 = local read "Re-SEC"() -> (w7204:bool)
                                n6751 = Or(x=w7203, y=w7204) -> (x .or. y?=w7202:bool)
                                n6752 = case shown="True" w7202 {
                                frame False {
                                }
                                frame True {
                                n6753 = local read "VISA Refnum in\nfor Pump"() -> (w7205:refnum<visa-resource-name>)
                                n6754 = call "HardStopCurrentProcess (SubVI).vi"("VISA Refnum in"=w7205) -> ()  [unwired: 11 in]
                                }
                                }
                                }
                                }
                                }
                                frame #2 {
                                # "Keeps the on-chip valve V1, V2 Open and V3 closed"
                                n6755 = while {
                                stop <- w7211 stop-if-true
                                n6756 = local read "Suction On/Off"() -> (w7212:bool)
                                n6757 = case shown="True" w7212 {
                                frame False {
                                n6758 = local read "Buffer-C2 Pumping\nResolution"() -> (w7218:T2)
                                n6759 = local read "Initial Plunger Position"() -> (w7217:dbl)
                                n6760 = local read "VISA Refnum in\nfor Pump"() -> (w7219:refnum<visa-resource-name>)
                                n6761 = local read "Position\nNow"() -> (w7215:dbl)
                                n6762 = local read "Volume of Syringe"() -> (w7216:dbl)
                                n6763 = local write "Volume being Injected \nin this process"(0.0) -> ()
                                n6764 = local write "Pause Data Collection"(FALSE) -> ()
                                n6765 = while {
                                tunnel: w7219 -> [w7226]
                                tunnel: w7218 -> [w7225]
                                tunnel: w7217 -> [w7221]
                                tunnel: w7216 -> [w7224]
                                tunnel: w7215 -> [w7220]
                                stop <- w7222 stop-if-true
                                n6766 = stacked-sequence {
                                tunnel: w7226 -> [w7232 w7254 w7279]
                                tunnel: w7225 -> [w7231 w7253 _]
                                tunnel: w7221 -> [w7229 _ _]
                                tunnel: w7224 -> [w7228 w7251 _]
                                tunnel: [_ _ w7271] -> w7222
                                tunnel: w7220 -> [_ w7249 _]
                                frame #0 {
                                # "From here on 'True Volume being injected \nin this process' represents the true total \nvolume in this process"
                                n6767 = call "AbsolutePlungerPosition (SubVI).vi"("VISA Refnum in"=w7232) -> ("Plunger Position"=w7230:i32)  [unwired: 10 in]
                                n6768 = case shown="..\"Standard Pumping\"" w7231 {
                                tunnel: w7230 -> [w7240 w7248]
                                tunnel: w7229 -> [w7239 w7247]
                                tunnel: w7228 -> [w7236 w7244]
                                tunnel: [w7233 w7241] -> w7227
                                frame .."Standard Pumping" {
                                n6769 = Subtract(x=w7240, y=w7239) -> (x-y=w7238:dbl)
                                n6770 = Absolute Value(x=w7238) -> (abs(x)=w7237:dbl)
                                n6771 = Multiply(x=w7237, y=w7236) -> (x*y=w7235:dbl)
                                n6772 = Divide(x=w7235, y=3000.0) -> (x/y=w7233:dbl)
                                }
                                frame "High Resolution Pumping".. {
                                n6773 = Subtract(x=w7248, y=w7247) -> (x-y=w7246:dbl)
                                n6774 = Absolute Value(x=w7246) -> (abs(x)=w7245:dbl)
                                n6775 = Multiply(x=w7245, y=w7244) -> (x*y=w7243:dbl)
                                n6776 = Divide(x=w7243, y=24000.0) -> (x/y=w7241:dbl)
                                }
                                }
                                n6777 = local write "True Volume being \ninjected in this\nprocess"(w7227) -> ()
                                }
                                frame #1 {
                                # "From here on 'Volume being injected \nin this process' represents the volume \nin this sub process"
                                n6778 = call "AbsolutePlungerPosition (SubVI).vi"("VISA Refnum in"=w7254) -> ("Plunger Position"=w7252:i32)  [unwired: 10 in]
                                n6779 = case shown="..\"Standard Pumping\"" w7253 {
                                tunnel: w7252 -> [w7262 w7270]
                                tunnel: w7249 -> [w7261 w7269]
                                tunnel: w7251 -> [w7258 w7266]
                                tunnel: [w7255 w7263] -> w7250
                                frame .."Standard Pumping" {
                                n6780 = Subtract(x=w7262, y=w7261) -> (x-y=w7260:dbl)
                                n6781 = Absolute Value(x=w7260) -> (abs(x)=w7259:dbl)
                                n6782 = Multiply(x=w7259, y=w7258) -> (x*y=w7257:dbl)
                                n6783 = Divide(x=w7257, y=3000.0) -> (x/y=w7255:dbl)
                                }
                                frame "High Resolution Pumping".. {
                                n6784 = Subtract(x=w7270, y=w7269) -> (x-y=w7268:dbl)
                                n6785 = Absolute Value(x=w7268) -> (abs(x)=w7267:dbl)
                                n6786 = Multiply(x=w7267, y=w7266) -> (x*y=w7265:dbl)
                                n6787 = Divide(x=w7265, y=24000.0) -> (x/y=w7263:dbl)
                                }
                                }
                                n6788 = local write "Volume being Injected \nin this process"(w7250) -> ()
                                }
                                frame #2 {
                                n6789 = local read "Stop for End of \nExperiment \nand Data Writing"() -> (w7274:bool)
                                n6790 = local read "Suction On/Off"() -> (w7275:bool)
                                n6791 = call "AbsolutePlungerPositionStatus (SubVI).vi"("VISA Refnum in"=w7279) -> ("read buffer"=w7278:string)  [unwired: 10 in]
                                n6792 = call <vilib>:"Trim Whitespace.vi"("string"=w7278) -> ("trimmed string"=w7277:string)  [unwired: 1 in]
                                n6793 = Equal?(x=w7277, y="/0`\u0003") -> (x = y?=w7273:bool)
                                n6794 = Or(x=w7275, y=w7274) -> (x .or. y?=w7272:bool)
                                n6795 = Or(x=w7273, y=w7272) -> (x .or. y?=w7271:bool)
                                }
                                }
                                n6796 = Wait (ms)(milliseconds to wait=u32 100) -> ()  [unwired: 1 out]
                                }
                                }
                                frame True {
                                n6797 = stacked-sequence {
                                frame #0 {
                                n6798 = local read "Suction Pressure\nfor EM-grid \nDeposition (mbar)"() -> (w7284:sgl)
                                n6799 = local write "Valve V4 Open"(FALSE ("Valve V4 Open")) -> ()
